vi "Release-errors.vi"(8 "error in (no error)":errorcluster, 11 "Data ref. in":refnum<data-value>) -> (0 "error out":errorcluster, 3 "Data ref.":refnum<data-value>)   [LabVIEW 2013, in "CameraVision.lvlib" / "CV-Main.lvclass"]
uses:
  CV-Main.lvclass
  CV-Main.lvclass/CV-Main.ctl
  Read Errors.vi
  Errors/CV-Errors.lvclass
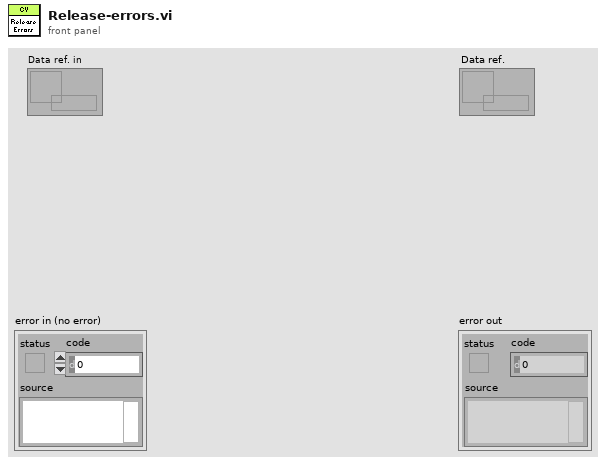
[diagram p1: front panel]
types:
  T1 = typedef "CameraVision.lvlib/CV-Errors.lvclass/Object-reference.ctl" = refnum<data-value>
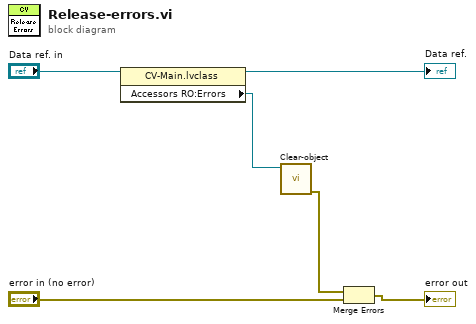
[diagram p0: block diagram]
diagram:
  n1 = property class="CV-Main.lvclass"(reference="Data ref. in") -> (reference out=→"Data ref.":refnum<data-value>, "Accessors RO:Errors"=w2:T1)  [unwired: 1 in, 1 out]
  n2 = call "Clear-object.vi"("Errors in"=w2) -> ("error out"=w6:errorcluster)  [unwired: 9 in, 1 out]
  n3 = Merge Errors(w6, "error in (no error)") -> (→"error out":errorcluster)
